vi "Reports.Result State to String.vi"(7 "Result State":T1 items=["LOG", "PASS", "FAIL", "ERROR"]) -> (3 "String Out":string)   [LabVIEW 2024]
uses:
  Results/Result.Measurement and Attribute Item Status.ctl
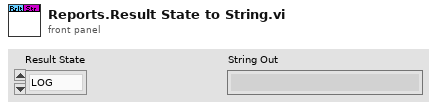
[diagram p1: front panel]
types:
  T1 = typedef "Result.Measurement and Attribute Item Status.ctl" = i32
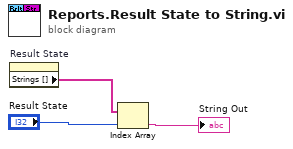
[diagram p0: block diagram]
diagram:
  n1 = property on="Result State" class="Ring (strict)"() -> ("Strings []"=w3:string[])  [unwired: 2 in, 2 out]
  n2 = Index Array(array=w3, index="Result State") -> (element=→"String Out":string)
